vi "Begin.vi"() -> (0 "error out":errorcluster)   [LabVIEW 2013]
doc: "Called before other user functions, this VI is expected to open initial I/O refnums, load in file data, and do all program initialization. Notice that the <B>error out</B> terminal is simply used for data flow. Wiring it to other structures or subVIs ensures that this VI runs first."
uses:
  <vilib>/Rock Robotics/WPI/DriverStation/WPI_DriverStationRobotMode2.ctl
  <vilib>/Rock Robotics/WPI/Joystick/WPI_JoystickDeviceEnum.ctl
  <vilib>/Rock Robotics/SystemInterfaces/DIO/FPGA_DIORelayChannel.ctl
  <vilib>/Rock Robotics/SystemInterfaces/DIO/FPGA_DIOChannel.ctl
  <vilib>/Rock Robotics/SystemInterfaces/Typedef/FPGA_TypedefDigitalModule.ctl
  <vilib>/Rock Robotics/WPI/Solenoid/WPI_SolenoidChannel.ctl
  <vilib>/Rock Robotics/SystemInterfaces/DIO/FPGA_DIOPWMChannel.ctl
  <vilib>/Rock Robotics/WPI/SafetyOutput/WPI_SafetyOutputConfigMenu.ctl
  TankDriveAction.ctl
  PnuematicMode.ctl
  <vilib>/Rock Robotics/WPI/Camera/WPI_CameraWhite Balance Values.ctl
  <vilib>/Rock Robotics/WPI/Camera/WPI_CameraExposure Values.ctl
  <vilib>/Rock Robotics/WPI/Camera/WPI_CameraFrameRate.ctl
  <vilib>/Rock Robotics/WPI/Camera/WPI_CameraImageSize.ctl
  Example_Code/Gyro/Read Angle Mode.ctl
  <vilib>/Rock Robotics/SystemInterfaces/Typedef/FPGA_TypedefAnalogModuleForGyro.ctl
  <vilib>/Rock Robotics/SystemInterfaces/AI/FPGA_AIGyroChannel.ctl
  Example_Code/Ultrasonic/SonarAction.ctl
  <vilib>/Rock Robotics/SystemInterfaces/Typedef/FPGA_TypedefAnalogModule.ctl
  <vilib>/Rock Robotics/SystemInterfaces/AI/FPGA_AIChannel.ctl
  Robot Global Data.vi
  <vilib>/Rock Robotics/WPI/Solenoid/WPI_SolenoidOpenSingle.vi
  <vilib>/Rock Robotics/WPI/RobotDrive/WPI_RobotDriveOpen4MotorWithTalon.vi
  ErrorTest/OutputError.vi
  <vilib>/Rock Robotics/WPI/Compressor/WPI_CompressorGetSetRefNum.vi
  <vilib>/Rock Robotics/WPI/Counter/WPI_CounterDigitalInputToDigitalSource.vi
  <vilib>/Rock Robotics/WPI/Encoder/WPI_EncoderType.ctl
panel:
  in  "UseQueue?":bool
  in  "Version":string="1.3.1"
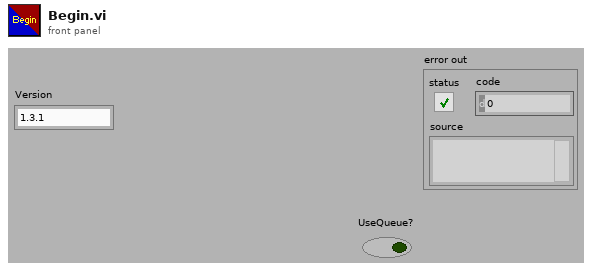
[diagram p1: front panel]
types:
  T1 = typedef "FPGA_AIChannel.ctl" = enum8{"AI 1", "AI 2", "AI 3", "AI 4", "AI 5", "AI 6", "AI 7", "AI 8", "Invalid"}
  T2 = typedef "FPGA_TypedefAnalogModule.ctl" = enum16{"Analog Module 1", "Analog Module 2"}
  T3 = typedef "SonarAction.ctl" = enum16{"Init", "ReadValue", "Disable"}
  T4 = typedef "FPGA_AIGyroChannel.ctl" = enum8{"AI 1", "AI 2", "Invalid"}
  T5 = typedef "FPGA_TypedefAnalogModuleForGyro.ctl" = enum16{"Analog Module 1"}
  T6 = typedef "Read Angle Mode.ctl" = enum16{"Init", "ReadAngle", "Disable"}
  T7 = typedef "WPI_CameraImageSize.ctl" = enum16{"640x480", "320x240", "160x120"}
  T8 = typedef "WPI_CameraFrameRate.ctl" = u32
  T9 = typedef "WPI_CameraExposure Values.ctl" = enum16{"Auto", "Flicker-free 50 Hz", "Flicker-free 60 Hz", "Hold current"}
  T10 = typedef "WPI_CameraWhite Balance Values.ctl" = enum16{"Auto", "Fixed indoor", "Fixed outdoor 1", "Fixed outdoor 2", "Fixed fluorescent 1", "Fixed fluorescent 2", "Hold current"}
  T11 = typedef "PnuematicMode.ctl" = enum16{"Init", "SetState", "Disable"}
  T12 = typedef "WPI_SolenoidChannel.ctl" = enum8{"Solenoid 1", "Solenoid 2", "Solenoid 3", "Solenoid 4", "Solenoid 5", "Solenoid 6", "Solenoid 7", "Solenoid 8", "Invalid"}
  T13 = typedef "FPGA_DIOPWMChannel.ctl" = enum8{"PWM 1", "PWM 2", "PWM 3", "PWM 4", "PWM 5", "PWM 6", "PWM 7", "PWM 8", "PWM 9", "PWM 10", "Invalid"}
  T14 = typedef "TankDriveAction.ctl" = enum16{"Init", "LinearDrive", "SetValue", "Disable"}
  T15 = typedef "WPI_SafetyOutputConfigMenu.ctl" = enum16{"Enable", "Disable"}
  T16 = typedef "FPGA_TypedefDigitalModule.ctl" = enum16{"Digital Module 1", "Digital Module 2"}
  T17 = typedef "FPGA_DIOChannel.ctl" = enum8{"DIO 1", "DIO 2", "DIO 3", "DIO 4", "DIO 5", "DIO 6", "DIO 7", "DIO 8", "DIO 9", "DIO 10", "DIO 11", "DIO 12", "DIO 13", "DIO 14", "Invalid"}
  T18 = typedef "FPGA_DIORelayChannel.ctl" = enum8{"Relay 1", "Relay 2", "Relay 3", "Relay 4", "Relay 5", "Relay 6", "Relay 7", "Relay 8", "Invalid"}
  T19 = typedef "WPI_JoystickDeviceEnum.ctl" = enum16{"USB 1", "USB 2", "USB 3", "USB 4", "Kinect 1", "Kinect 2"}
  T20 = typedef "WPI_DriverStationRobotMode2.ctl" = enum16{"Autonomous Disabled", "Autonomous Enabled", "Teleop Disabled", "Teleop Enabled", "Timeout", "Finish", "Test Disabled", "Test Enabled"}
  T21 = typedef "WPI_EncoderType.ctl" = enum16{"1x", "2x", "4x"}
  T22 = typedef "WPI_DigitalInputDevRef.ctl" = cluster{"DevStatus":errorcluster, "DIO Channel":T17, "Digital Module":T16}
  T23 = typedef "FPGA_CounterEncoderSourceConvertionLVSourceType.ctl" = cluster{"DevStatus":errorcluster, "AnalogTriggerMode?":bool, "DigitalMode":cluster{"Digital Module":T16, "DIO Channel":T24}, "AnalogTriggerMode":cluster{"AnalogTriggerIndex":T25, "OutputType":T26}}
  T24 = typedef "FPGA_DIODigitalSourceChannel.ctl" = enum8{"DIO 1", "DIO 2", "DIO 3", "DIO 4", "DIO 5", "DIO 6", "DIO 7", "DIO 8", "DIO 9", "DIO 10", "DIO 11", "DIO 12", "DIO 13", "DIO 14", "Disabled"}
  T25 = typedef "FPGA_AnalogTriggerIndex.ctl" = enum8{"Trig 0", "Trig 1", "Trig 2", "Trig 3", "Trig 4", "Trig 5", "Trig 6", "Trig 7", "Invalid"}
  T26 = typedef "FPGA_AnalogTriggerOutType.ctl" = enum16{"InWindow", "TriggerState", "Rising", "Falling"}
  T27 = typedef "WPI_EncoderDevRef.ctl" = cluster{"DevStatus":errorcluster, "EncoderIndex":T28, "CounterIndex":T29, "DistancePerCount":dbl, "Decoding Type":T21}
  T28 = typedef "FPGA_EncoderIdx.ctl" = enum8{"Enc 0", "Enc 1", "Enc 2", "Enc 3", "Invalid"}
  T29 = typedef "FPGA_CounterCtrSystemIndex.ctl" = enum8{"Ctr 0", "Ctr 1", "Ctr 2", "Ctr 3", "Ctr 4", "Ctr 5", "Ctr 6", "Ctr 7", "Invalid"}
  T30 = typedef "WPI_SolenoidDevRef.ctl" = cluster{"DevStatus":errorcluster, "Solenoid Module":T31, "Forward Solenoid Channel":T12, "Reverse Solenoid Channel":T12}
  T31 = typedef "FPGA_TypedefSolenoidModule.ctl" = enum16{"Solenoid Module 1", "Solenoid Module 2"}
  T32 = typedef "WPI_GyroDevRef.ctl" = cluster{"DevStatus":errorcluster, "Analog Module":T2, "Analog Channel":T1, "Offset":dbl, "Gain (VoltsPerDegree/Second)":dbl}
  T33 = typedef "WPI_AnalogChannelDevRef.ctl" = cluster{"DevStatus":errorcluster, "Analog Module":T2, "Analog Channel":T1}
  T34 = typedef "WPI_RobotDriveDevRef.ctl" = cluster{"DevStatus":errorcluster, "Motors[]":T35[], "Square Inputs":bool, "Max Output":dbl, "Isochronous":bool}
  T35 = typedef "WPI_MotorControlDeviceRef.ctl" = cluster{"DeviceStatus":errorcluster, "Type":enum16{"PWM", "CAN"}, "PWM":cluster{"Digital Module":T16, "PWM Channel":T13, "DeadBand":T36}, "CAN":cluster{"Device Number":u8, "Control Mode":T37, "Semaphore":T38, "Max Vout":dbl}, "Invert":bool, "TransformRef":T39, "InvTransformRef":T39}
  T36 = typedef "WPI_PWMDeadband.ctl" = cluster{"Name":string, "maxPositivePwm":i32, "minPositivePwm":i32, "centerPwm":i32, "maxNegativePwm":i32, "minNegativePwm":i32, "angularRange":u16}
  T37 = typedef "WPI_CANJaguar_ControlMode.ctl" = enum8{"Percent VBus", "Current", "Speed", "Position", "Voltage"}
  T38 = typedef "Semaphore RefNum" = refnum<k1>
  T39 = typedef "WPI_PWMTransform_ConPane.ctl" = refnum<vi>
  T40 = typedef "WPI_CameraDevRef.ctl" = cluster{"Camera Address":string, "CameraStatus":errorcluster, "Acquire Image Notifier":refnum<notifier>}
  T41 = typedef "WPI_JoystickDevRef.ctl" = cluster{"Device":T19}
  T42 = typedef "WPI_CompressorDevRef.ctl" = cluster{"DevStatus":errorcluster, "DigitalInputDevRef":T22, "RelayDevRef":T43}
  T43 = typedef "WPI_RelayDevRef.ctl" = cluster{"DevStatus":errorcluster, "Relay Channel":T18, "Digital Module":T16, "Relay Direction":T44}
  T44 = typedef "WPI_RelayDirection.ctl" = enum16{"Both directions", "Forward only", "Reverse only"}
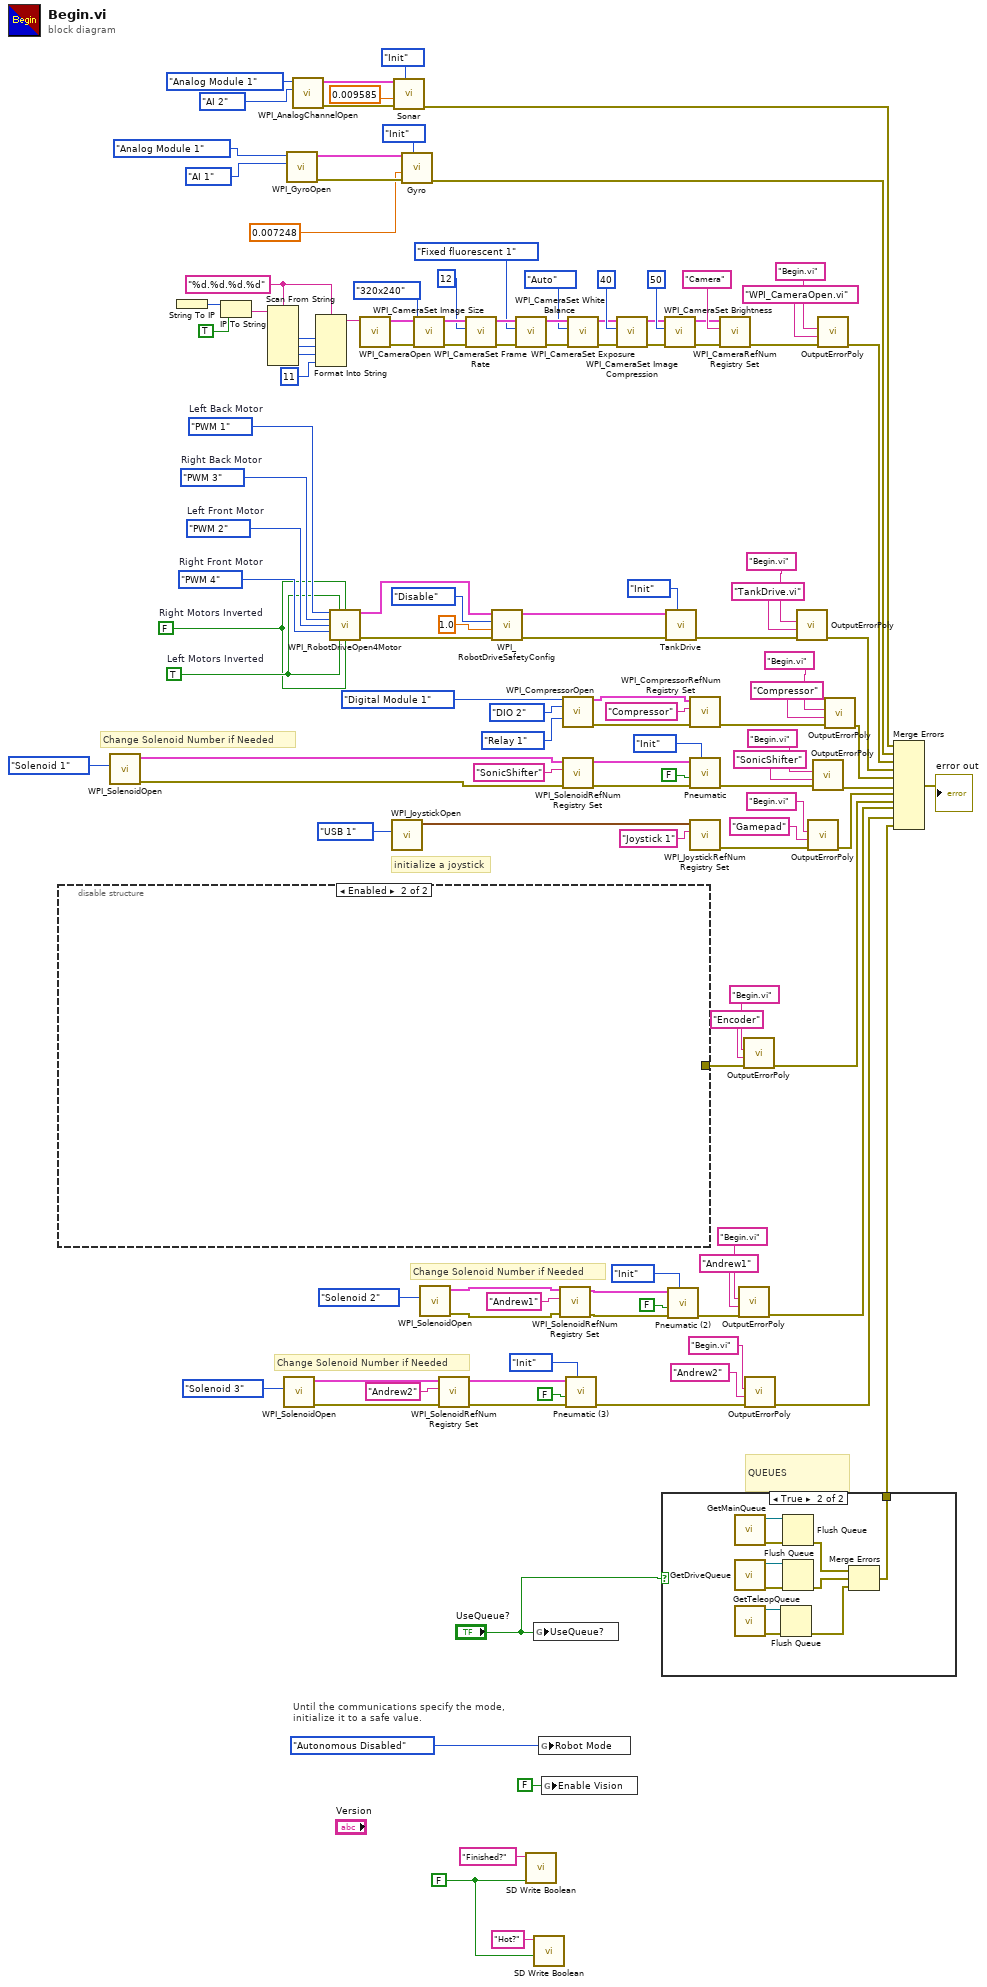
[diagram p0: block diagram]
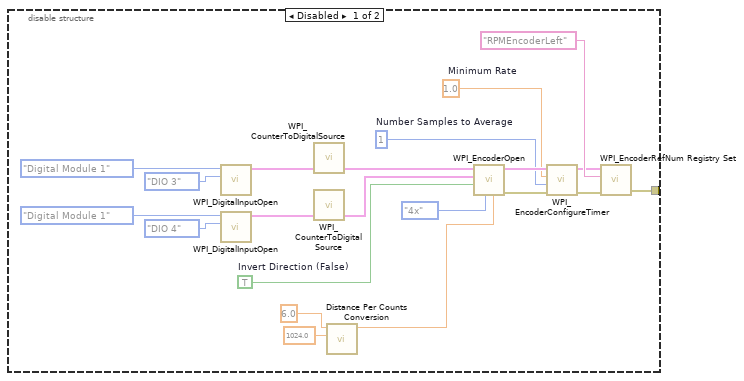
[diagram p3: hidden frame]
diagram:
  w6 = FALSE ("Boolean")
  w58 = "%d.%d.%d.%d" ("format string")
  w110 = FPGA_DIOPWMChannel."PWM 4"  # Right Front Motor
  w111 = FPGA_DIOPWMChannel."PWM 2"  # Left Front Motor
  w116 = FPGA_DIOPWMChannel."PWM 3"  # Right Back Motor
  w117 = FPGA_DIOPWMChannel."PWM 1"  # Left Back Motor
  w108 = FALSE  # Right Motors Inverted
  w109 = TRUE  # Left Motors Inverted
  # "QUEUES"
  # "Change Solenoid Number if Needed"
  # "Change Solenoid Number if Needed"
  # "Change Solenoid Number if Needed"
  # "initialize a joystick"
  # "Until the communications specify the mode,\ninitialize it to a safe value."
  n1 = disable-structure shown="Enabled" {
    disable-tunnel: [w131 _] -> w40
    frame Disabled {
      w138 = TRUE  # Invert Direction (False)
      w140 = u8 1  # Number Samples to Average
      w141 = 1.0  # Minimum Rate
      n2 = call <vilib>:"WPI_DigitalInputOpen.vi"("DIO Channel"=FPGA_DIOChannel."DIO 3", "Digital Module (Module 1)"=FPGA_TypedefDigitalModule."Digital Module 1") -> ("DigitalInputDevRef"=w148:T22)  [unwired: 1 in, 8 out]
      n3 = call <vilib>:"WPI_DigitalInputOpen.vi"("DIO Channel"=FPGA_DIOChannel."DIO 4", "Digital Module (Module 1)"=FPGA_TypedefDigitalModule."Digital Module 1") -> ("DigitalInputDevRef"=w149:T22)  [unwired: 1 in, 8 out]
      n4 = call-poly <vilib>:"WPI_CounterToDigitalSource.vi"("DigitalInputDevRef"=w148) -> ("Digital Source"=w147:T23)  [unwired: 6 out]
      n5 = call-poly <vilib>:"WPI_CounterToDigitalSource.vi"("DigitalInputDevRef"=w149) -> ("Digital Source"=w150:T23)  [unwired: 6 out]
      n6 = call "Distance Per Counts Conversion.vi"("Counts Per Rev"=1024.0, "WheelDiameter"=6.0) -> ("Distance/Count"=w134:dbl)  [unwired: 9 in]
      n7 = call <vilib>:"WPI_EncoderOpen.vi"("DistancePerCount"=w134, "Decoding Type"=WPI_EncoderType."4x", "Invert Direction (False)"=w138, "BSource"=w150, "ASource"=w147) -> ("error out"=w136:errorcluster, "EncoderDevRef"=w144:T27)  [unwired: 3 in, 2 out]
      n8 = call <vilib>:"WPI_EncoderConfigureTimer.vi"("error in (no error)"=w136, "Number Samples to Average"=w140, "Minimum Rate"=w141, "EncoderDevRef"=w144) -> ("error out"=w135:errorcluster, "EncoderDevRef"=w137:T27)  [unwired: 6 out]
      n9 = call <vilib>:"WPI_EncoderRefNum Registry Set.vi"("error in (no error)"=w135, "refnum name"="RPMEncoderLeft", "EncoderDevRef"=w137) -> ("error out"=w131:errorcluster)  [unwired: 7 in, 1 out]
    }
    frame Enabled {
    }
  }
  n10 = call-poly <vilib>:"WPI_SolenoidOpen.vi"("Solenoid Channel"=WPI_SolenoidChannel."Solenoid 1") -> ("error out"=w118:errorcluster, "SolenoidDevRef"=w120:T30)  [unwired: 9 in]
  n11 = String To IP() -> (0:w65:u32)  [unwired: 1 in]
  n12 = IP To String(1:TRUE ("dot notation? (F)"), 2:w65) -> (0:w63:string)
  n13 = Scan From String(format string=w58, input string=w63) -> (output 1=w62:i32, output 2=w61:i32, output 3=w60:i32)  [unwired: 7 in, 3 out]
  n14 = call-poly <vilib>:"WPI_SolenoidOpen.vi"("Solenoid Channel"=WPI_SolenoidChannel."Solenoid 3") -> ("error out"=w99:errorcluster, "SolenoidDevRef"=w100:T30)  [unwired: 9 in]
  n15 = call <vilib>:"WPI_GyroOpen.vi"("Analog Channel"=FPGA_AIGyroChannel."AI 1" ("Channel 2"), "Analog Module (Module 1)"=FPGA_TypedefAnalogModuleForGyro."Analog Module 1" ("Analog Module 2")) -> ("error out"=w3:errorcluster, "GyroDevRef"=w2:T32)  [unwired: 4 in, 4 out]
  n16 = call <vilib>:"WPI_AnalogChannelOpen.vi"("Analog Channel"=FPGA_AIChannel."AI 2", "Analog Module (Module 1)"=FPGA_TypedefAnalogModule."Analog Module 1") -> ("error out"=w13:errorcluster, "AIDeviceRef"=w14:T33)  [unwired: 8 in]
  n17 = Format Into String(format string=w58, w62, w61, w60, 11 ("Compression")) -> (resulting string=w57:string)  [unwired: 2 in, 1 out]
  n18 = call-poly <vilib>:"WPI_RobotDriveOpen4Motor.vi"("Rear Left Motor"=w117, "Rear Left Motor Inverted"=w109, "Rear Right Motor Inverted"=w108, "Rear Right Motor"=w116, "Front Left Motor"=w111, "Front Right Motor"=w110, "Front Left Motor Inverted"=w109, "Front Right Motor Inverted"=w108) -> ("RobotDriveDevRef"=w115:T34, "error out"=w114:errorcluster)  [unwired: 6 in]
  n19 = call <vilib>:"WPI_CameraOpen.vi"("Camera Address"=w57) -> ("error out"=w76:errorcluster, "CameraDevRef"=w77:T40)  [unwired: 1 in, 8 out]
  n20 = call <vilib>:"WPI_JoystickOpen.vi"("JoystickDevice"=WPI_JoystickDeviceEnum."USB 1") -> ("JoystickDevRef"=w128:T41)  [unwired: 10 in]
  n21 = call "Sonar.vi"("Action"=SonarAction."Init", "error in (no error)"=w13, "Scaling factor (V/in)"=0.009585, "AIDeviceRef"=w14) -> ("error out"=w9:errorcluster)  [unwired: 6 in, 1 out]
  n22 = call "Gyro.vi"("Action"=Read_Angle_Mode."Init" ("Enum"), "error in"=w3, "Gain (VoltsPerDegree/Second)"=0.007248, "GyroDevRef"=w2) -> ("error out"=w19:errorcluster)  [unwired: 6 in, 1 out]
  n23 = call <vilib>:"WPI_CameraSet Image Size.vi"("error in (no error)"=w76, "Image Size"=WPI_CameraImageSize."320x240", "CameraDevRef"=w77) -> ("error out"=w75:errorcluster, "CameraDevRef Out"=w78:T40)  [unwired: 7 out]
  n24 = call-poly <vilib>:"WPI_SolenoidOpen.vi"("Solenoid Channel"=WPI_SolenoidChannel."Solenoid 2") -> ("error out"=w102:errorcluster, "SolenoidDevRef"=w104:T30)  [unwired: 9 in]
  n25 = call <vilib>:"WPI_SolenoidRefNum Registry Set.vi"("error in (no error)"=w99, "refnum name"="Andrew2", "SolenoidDevRef"=w100) -> ("error out"=w91:errorcluster, "SolenoidDevRef"=w90:T30)  [unwired: 7 in]
  n26 = call <vilib>:"WPI_CameraSet Frame Rate.vi"("error in (no error)"=w75, "Frame Rate (fps)"=T8 12, "CameraDevRef"=w78) -> ("error out"=w74:errorcluster, "CameraDevRef Out"=w80:T40)  [unwired: 7 out]
  n27 = call <vilib>:"WPI_RobotDriveSafetyConfig.vi"("error in (no error)"=w114, "timeout (s)"=1.0, "mode"=WPI_SafetyOutputConfigMenu."Disable", "RobotDriveDevRef"=w115) -> ("error out"=w53:errorcluster, "RobotDriveDevRef"=w52:T34)  [unwired: 6 in]
  n28 = call <vilib>:"WPI_CameraSet White Balance.vi"("error in (no error)"=w74, "White Balance"=WPI_CameraWhite_Balance_Values."Fixed fluorescent 1", "CameraDevRef"=w80) -> ("error out"=w73:errorcluster, "CameraDevRef Out"=w79:T40)  [unwired: 7 out]
  n29 = call <vilib>:"SD Write Boolean.vi"("Boolean"=w6, "Name"="Finished?") -> ()  [unwired: 8 in, 2 out]
  n30 = global write "Robot Global Data.vi" "UseQueue?"("UseQueue?") -> ()
  n31 = call <vilib>:"SD Write Boolean.vi"("Boolean"=w6, "Name"="Hot?") -> ()  [unwired: 8 in, 2 out]
  n32 = global write "Robot Global Data.vi" "Robot Mode"(WPI_DriverStationRobotMode2."Autonomous Disabled" ("Robot Mode")) -> ()
  n33 = global write "Robot Global Data.vi" "Enable Vision"(FALSE ("Enable Vision")) -> ()
  n34 = call <vilib>:"WPI_SolenoidRefNum Registry Set.vi"("error in (no error)"=w102, "refnum name"="Andrew1", "SolenoidDevRef"=w104) -> ("error out"=w94:errorcluster, "SolenoidDevRef"=w95:T30)  [unwired: 7 in]
  n35 = call <vilib>:"WPI_CompressorOpen.vi"("Pressure Switch Digital Module (Module 1)"=FPGA_TypedefDigitalModule."Digital Module 1" ("Pressure Switch\nand Relay Module"), "Pressure Switch DIO Channel"=FPGA_DIOChannel."DIO 2" ("Pressure Switch Channel"), "Relay Channel"=FPGA_DIORelayChannel."Relay 1") -> ("CompressorDevRef"=w123:T42, "error out"=w107:errorcluster)  [unwired: 2 in, 9 out]
  n36 = call <vilib>:"WPI_SolenoidRefNum Registry Set.vi"("error in (no error)"=w118, "refnum name"="SonicShifter", "SolenoidDevRef"=w120) -> ("error out"=w97:errorcluster, "SolenoidDevRef"=w98:T30)  [unwired: 7 in]
  n37 = call "Pneumatic (3).vi"("Mode"=PnuematicMode."Init", "error in (no error)"=w91, "Default Position"=FALSE, "SolenoidDevRef"=w90) -> ("error out"=w36:errorcluster)  [unwired: 7 in]
  n38 = call <vilib>:"WPI_CameraSet Exposure.vi"("error in (no error)"=w73, "Exposure"=WPI_CameraExposure_Values."Auto", "CameraDevRef"=w79) -> ("error out"=w72:errorcluster, "CameraDevRef Out"=w82:T40)  [unwired: 7 out]
  n39 = call <vilib>:"WPI_CameraSet Image Compression.vi"("error in (no error)"=w72, "Compression"=40, "CameraDevRef"=w82) -> ("error out"=w71:errorcluster, "CameraDevRef Out"=w81:T40)  [unwired: 7 out]
  n40 = case shown="True" "UseQueue?" {
    tunnel: [_ w155] -> w17
    frame False {
    }
    frame True {
      n41 = call "GetMainQueue.vi"() -> ("error out"=w161:errorcluster, "queue out"=w160:refnum<queue>)  [unwired: 10 in]
      n42 = call "GetDriveQueue.vi"() -> ("error out"=w159:errorcluster, "queue out"=w158:refnum<queue>)  [unwired: 10 in]
      n43 = call "GetTeleopQueue.vi"() -> ("error out"=w154:errorcluster, "queue out"=w152:refnum<queue>)  [unwired: 10 in]
      n44 = Flush Queue(queue=w152, error in (no error)=w154) -> (error out=w153:errorcluster)  [unwired: 2 out]
      n45 = Flush Queue(queue=w160, error in (no error)=w161) -> (error out=w157:errorcluster)  [unwired: 2 out]
      n46 = Flush Queue(queue=w158, error in (no error)=w159) -> (error out=w156:errorcluster)  [unwired: 2 out]
      n47 = Merge Errors(w157, w156, w153) -> (w155:errorcluster)
    }
  }
  n48 = call <vilib>:"WPI_CameraSet Brightness.vi"("error in (no error)"=w71, "Brightness"=50, "CameraDevRef"=w81) -> ("error out"=w69:errorcluster, "CameraDevRef Out"=w70:T40)  [unwired: 7 out]
  n49 = call "TankDrive.vi"("DriveAction"=TankDriveAction."Init" ("Enum"), "error in (no error)"=w53, "RobotDriveDevRef"=w52) -> ("error out"=w48:errorcluster)  [unwired: 8 in]
  n50 = call "Pneumatic (2).vi"("Mode"=PnuematicMode."Init", "error in (no error)"=w94, "Default Position"=FALSE, "SolenoidDevRef"=w95) -> ("error out"=w38:errorcluster)  [unwired: 7 in]
  n51 = call <vilib>:"WPI_CompressorRefNum Registry Set.vi"("error in (no error)"=w107, "refnum name"="Compressor", "CompressorDevRef"=w123) -> ("error out"=w46:errorcluster)  [unwired: 7 in, 1 out]
  n52 = call "Pneumatic.vi"("Mode"=PnuematicMode."Init", "error in (no error)"=w97, "Default Position"=FALSE, "SolenoidDevRef"=w98) -> ("error out"=w44:errorcluster)  [unwired: 7 in]
  n53 = call <vilib>:"WPI_JoystickRefNum Registry Set.vi"("refnum name"="Joystick 1", "JoystickDevRef"=w128) -> ("error out"=w42:errorcluster)  [unwired: 8 in, 1 out]
  n54 = call <vilib>:"WPI_CameraRefNum Registry Set.vi"("error in (no error)"=w69, "refnum name"="Camera", "CameraDevRef"=w70) -> ("error out"=w56:errorcluster)  [unwired: 8 out]
  n55 = call-poly "OutputErrorPoly.vi"("error in (no error)"=w38, "Causing VI"="Andrew1" ("Calling VI"), "Calling VI"="Begin.vi") -> ("error out"=w37:errorcluster)  [unwired: 8 in]
  n56 = call-poly "OutputErrorPoly.vi"("error in (no error)"=w40, "Causing VI"="Encoder" ("Calling VI"), "Calling VI"="Begin.vi") -> ("error out"=w39:errorcluster)  [unwired: 8 in]
  n57 = call-poly "OutputErrorPoly.vi"("error in (no error)"=w36, "Causing VI"="Andrew2" ("Calling VI"), "Calling VI"="Begin.vi") -> ("error out"=w35:errorcluster)  [unwired: 8 in]
  n58 = call-poly "OutputErrorPoly.vi"("error in (no error)"=w48, "Causing VI"="TankDrive.vi" ("Calling VI"), "Calling VI"="Begin.vi") -> ("error out"=w47:errorcluster)  [unwired: 8 in]
  n59 = call-poly "OutputErrorPoly.vi"("error in (no error)"=w42, "Causing VI"="Gamepad" ("Calling VI"), "Calling VI"="Begin.vi") -> ("error out"=w41:errorcluster)  [unwired: 8 in]
  n60 = call-poly "OutputErrorPoly.vi"("error in (no error)"=w44, "Causing VI"="SonicShifter" ("Calling VI"), "Calling VI"="Begin.vi") -> ("error out"=w43:errorcluster)  [unwired: 8 in]
  n61 = call-poly "OutputErrorPoly.vi"("error in (no error)"=w56, "Causing VI"="WPI_CameraOpen.vi" ("Calling VI"), "Calling VI"="Begin.vi") -> ("error out"=w18:errorcluster)  [unwired: 8 in]
  n62 = call-poly "OutputErrorPoly.vi"("error in (no error)"=w46, "Causing VI"="Compressor" ("Calling VI"), "Calling VI"="Begin.vi") -> ("error out"=w45:errorcluster)  [unwired: 8 in]
  n63 = Merge Errors(w9, w19, w18, w47, w45, w43, w41, w39, w37, w35, w17) -> (→"error out":errorcluster)
